vi "Read Measurement (Time Interval Error).vi"(0 "VISA resource name":refnum<visa-resource-name>, 1 "Direction (0: Rising)":i32(ring) items=["Rising", "Falling", "Both"], 2 "Units (0: Second)":i32(ring) items=["Second", "Unit Interval"], 5 "Channel (1: Channel 1)":u16(ring) items=["Channel 1", "Channel 2", "Channel 3", "Channel 4", "Function 1", "Function 2", "Function 3", "Function 4", "Memory 1", "Memory 2", "Memory 3", "Memory 4"], 7 "Measurement Function (0: Time Interval Error (Data))":i32(ring) items=["Time Interval Error (Data)", "Time Interval Error (Clock)"], 9 "Maximum Time (10000ms)":u32, 11 "error in (no error)":errorcluster) -> (4 "VISA resource name out":refnum<visa-resource-name>, 6 "Time Interval Error(s)":dbl, 15 "error out":errorcluster)   [LabVIEW 2009, in "Agilent 8000 Series.lvlib"]
doc: "Measures the time interval error on a clock or data time interval error. \n\nThis VI initiates an acquisition on the channel that the end-user defines. It then waits for the acquisition to complete, obtains a waveform measurement on the channel the end-user specifies, and returns the measurement value."
uses:
  Agilent 8000 Series.lvlib
  Low Level/Fetch Measurement (Time Interval Error).vi
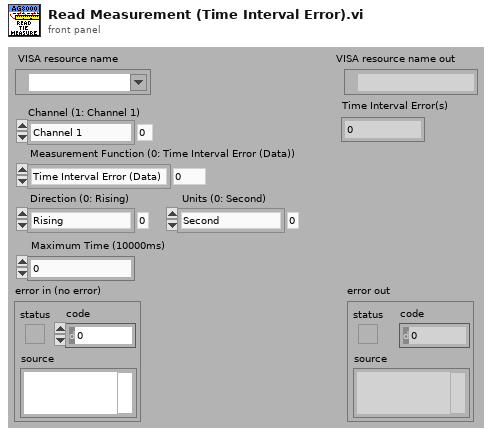
[diagram p1: front panel]
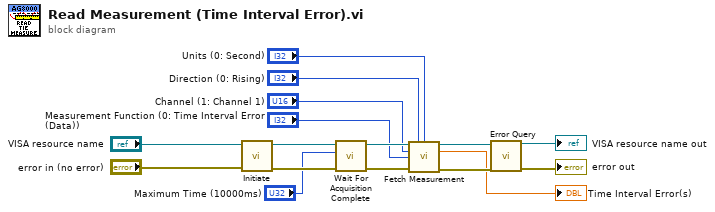
[diagram p0: block diagram]
diagram:
  n1 = call "Initiate.vi"("error in (no error)"="error in (no error)", "VISA resource name"="VISA resource name") -> ("error out"=w9:errorcluster, "VISA resource name out"=w10:refnum<visa-resource-name>)  [unwired: 8 in]
  n2 = call "Wait For Acquisition Complete.vi"("error in (no error)"=w9, "Maximum Time (10000ms)"="Maximum Time (10000ms)", "VISA resource name"=w10) -> ("error out"=w11:errorcluster, "VISA resource name out"=w12:refnum<visa-resource-name>)  [unwired: 7 in]
  n3 = call-poly "Fetch Measurement.vi"("VISA resource name"=w12, "Direction (0: Rising)"="Direction (0: Rising)", "Units (0: Second)"="Units (0: Second)", "Channel (1: Channel 1)"="Channel (1: Channel 1)", "Measurement Function (0: Time Interval Error (Data))"="Measurement Function (0: Time Interval Error (Data))", "error in (no error)"=w11) -> ("VISA resource name out"=w7:refnum<visa-resource-name>, "Time Interval Error (s)"=→"Time Interval Error(s)":dbl, "error out"=w8:errorcluster)  [unwired: 7 in]
  n4 = call "Error Query.vi"("error in (no error)"=w8, "VISA resource name"=w7) -> ("error out"=→"error out":errorcluster, "VISA resource name out"=→"VISA resource name out":refnum<visa-resource-name>)  [unwired: 6 in, 2 out]
